vi "TestStand - Initialize Property Value_1D Array.vi"(0 "Sequence Context":refnum<k7>, 2 "Lookup String":string="Locals.NumericArray", 5 "Data In":dbl[](array[numeric]), 11 "Error In":errorcluster) -> (15 "Error Out":errorcluster)   [LabVIEW 2013]
doc: "This VI inserts 1D array into TestStand 1D Array"
uses:
  <vilib>/addons/TestStand/_TSUtility.llb/TestStand - Set Property Value (Numeric Array).vi
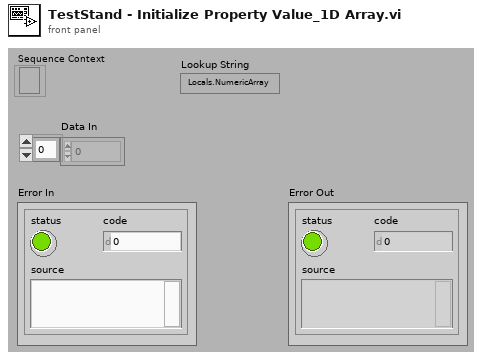
[diagram p1: front panel]
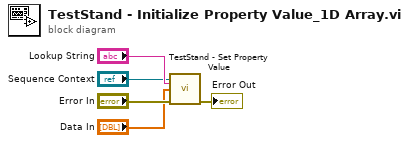
[diagram p0: block diagram]
diagram:
  n1 = call-poly <vilib>:"TestStand - Set Property Value.vi"("Sequence Context In"="Sequence Context", "Lookup String"="Lookup String", "New Value"="Data In", "error in (no error)"="Error In") -> ("error out"=→"Error Out":errorcluster)  [unwired: 1 in, 10 out]
